vi "LaserMaster.vi"() -> ()   [LabVIEW 2013]
uses:
  <vilib>/Instr/_visa.llb/VISA Configure Serial Port (Instr).vi
  <vilib>/Utility/file.llb/Write To Spreadsheet File (string).vi
panel:
  out "Humidity Threshold":dbl
  in  "Power (mW) 2":dbl format="%#.0f"
  out "SavePath":path
  out "Start time":timestamp
  out "Step":dbl
  out "State next step":string
  in  "stop":bool
  out "Query backup List":string[][](array[string])=[["?L", " 0\r"], ["?K", " 0\r"], ["?F", " 0\r"], ["?FH", " 2\r"], ["?SHUTTER", " 0\r"], ["?UF", " 0\r"], ["?PHLDC", " 1\r"], ["?PZTMC", " 0\r"], ["?PZTXC", " 2.24\r"], ["?PZTYC", " 2.14\r"], ["?PHLDP", " 0\r"], ["?PZTMP", " 0\r"], ["?PZTXP", " 2.58\r"], ["?PXTYP", "  Query Error:?PXTYP\r"], ["?PTRK", "  Query Error:?PTRK\r"], ["?MDLK", " 0\r"], ["?PP", " 0.80\r"], ["?TS", " 0\r"], ["?SM", " 1\r"], ["?HM", " 1\r"], ["?VW", " 850\r"], ["?STPRPOS", " 2096\r"], ["?C", " 0.00\r"], ["?D1C", " 0.08\r"], ["?D2C", " -0.43\r"], ["?BT", " 20.07\r"], ["?D1T", " 24.20\r"], ["?D2T", " 24.20\r"], ["?VT", " 20.72\r"], ["?LBOT", " 148.45\r"], ["?ET", " 39.01\r"], ["?D1ST", " 24.20\r"], ["?D2ST", " 24.20\r"], ["?VST", " 30.00\r"], ["?LBOST", " 148.41\r"], ["?EST", " 39.00\r"], ["?D1TD", " 500.12\r"], ["?D2TD", " 464.53\r"], ["?VD", " 0.00\r"], ["?LBOD", " 5358.08\r"], ["?ED", " 2152.46\r"], ["?D1HST", " 21.35\r"], ["?D2HST", " 21.48\r"], ["?LBOH", " 1\r"], ["?LRS", " 2\r"], ["?D1SS", " 1\r"], ["?D2SS", " 1\r"], ["?VSS", " 0\r"], ["?LBOSS", " 1\r"], ["?ESS", " 1\r"], ["?D1H", "  351.54\r"], ["?D2H", "  351.52\r"], ["?HH", " 37\r"], ["?D1V", " 0.19\r"], ["?D2V", " 0.18\r"], ["?SV", " 8.26,8.26,9.57\r"], ["?MB", "  Query Error:?MB\r"], ["?PI", " 2BC\r"], ["?BV", " 13.24\r"], ["?AMDLK", " 1\r"], ["?PZTS", "  Query Error:?PZTS\r"], ["?TMAX", " 1080\r"], ["?TMIN", " 680\r"], ["?ALIGN", " 0\r"], ["?ALIGNP", " 250\r"], ["?ALIGNW", " 730\r"], ["?LFP", " 0\r"], ["?PZTXCM", " 8.11\r"], ["?PZTXCP", " -10.30\r"], ["?PZTXPM", " 8.11\r"], ["?PZTXPP", " 3.06\r"], ["?PZTYCM", " 8.11\r"], ["?PZTYCP", " -14.28\r"], ["?PZTYPM", " 8.11\r"], ["?PZTYPP", " 11.74\r"], ["?RH", " 0\r"], ["?SN", " 9571\r"], ["?ST", " Standby\r"], ["?GDDCURVE", " 0\r"], ["?GDD", " 0\r"], ["?GDDCURVEN", " ZERO\r"], ["?CURVEN", " OUT OF RANGE\r"], ["?COMP", " 1\r"], ["?HMCOMP", " 1\r"], ["?GDDMAX", " 17333\r"], ["?GDDMIN", "0"]]
  out "Laser Info":i32
  out "Shutter off time":dbl
  out "Quiting":dbl
  out "Backuper state":string
  in  "Tab Control":T1(tab)
  in  "Auto":bool
  out "Baseplate Temp (C)":dbl(slide) scale=20.0..40.0
  in  "Dither hold":bool
  in  "Shutter":bool
  in  "Lock":bool
  out "Laser Status":bool
  out "Power (mW)":dbl(knob) scale=0.0..5000.0
  out "Walking":bool
  out "Sleeping":bool
  out "ModeLocked":bool
  out "Backing up":bool
  in  "Wavelength":dbl
  in  "GDD":dbl
  in  "Align":bool
  in  "QUIT":bool
  out "Max":string
  in  "Dither auto":dbl=120.0
  in  "Dither timer":dbl=5.0
  out "Faults":string
  in  "Home motor":bool
  in  "Optimize":bool
  in  "WV Walk":bool
  in  "Auto-Standby\nTime (min)":dbl=120.0
  in  "Sleep":bool
  in  "Backup":bool
  in  "Auto-Backup \nIdle Time (min)":dbl=30.0
  out "Operating Status":string
  out "Tunning Status":i32
  out "Idle Time":dbl format="%.1f"
  out "Laser On Time":dbl format="%#.1f"
  in  "Laser Control":bool
  in  "Command Line":string
  out "Laser Response":string
  in  "Refresh":bool
  out "Query List":string[][](array[string])
  out "queue #":i32
  # "LASER"
  # "LASER fine-tune"
  # "BACKUP"
  # "Timers"
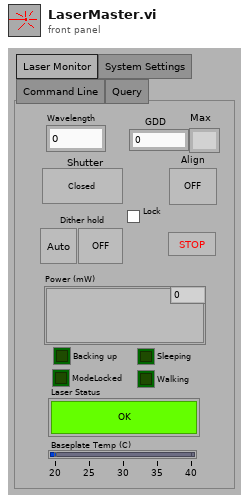
[diagram p1: front panel]
types:
  T1 = enum32{"Laser Monitor", "System Settings", "Command Line", "Query"}
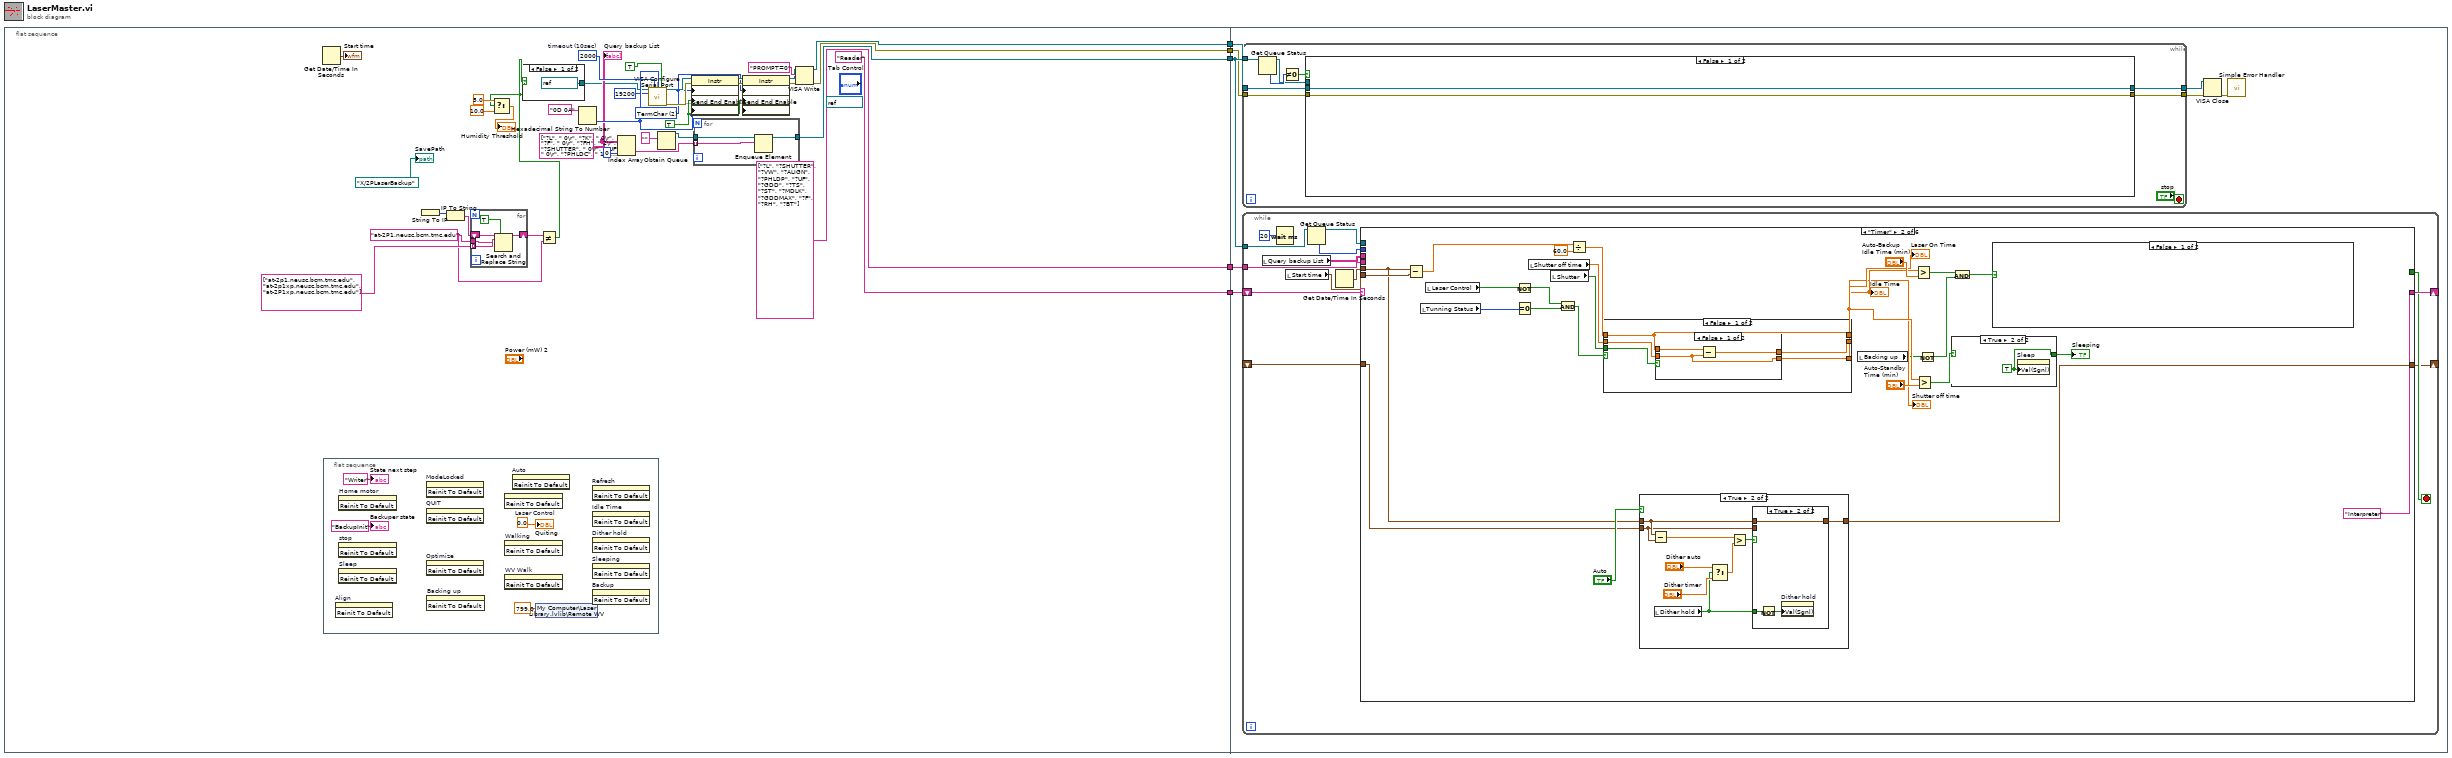
[diagram p0: block diagram]
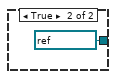
[diagram p2: hidden frame]
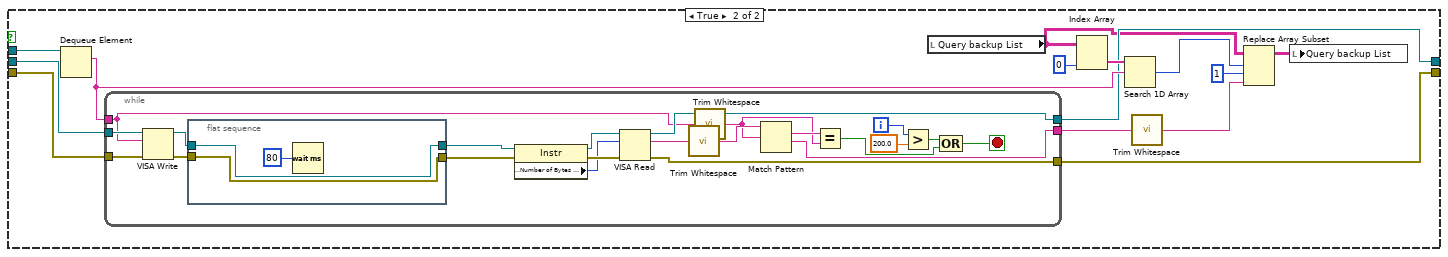
[diagram p3: hidden frame]
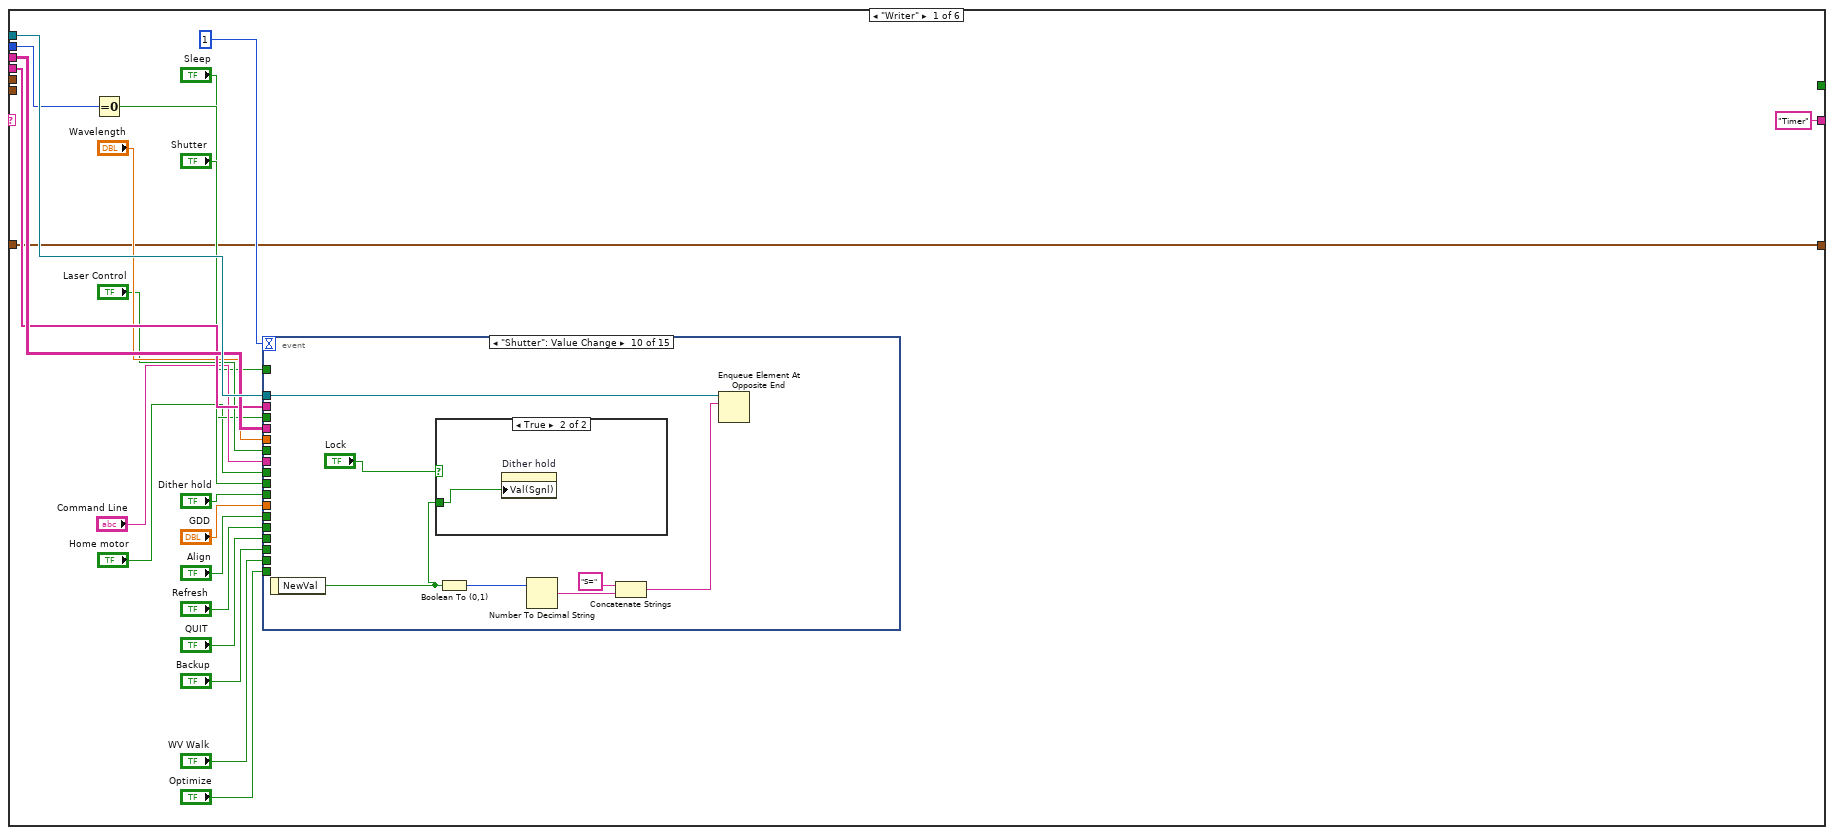
[diagram p4: hidden frame]
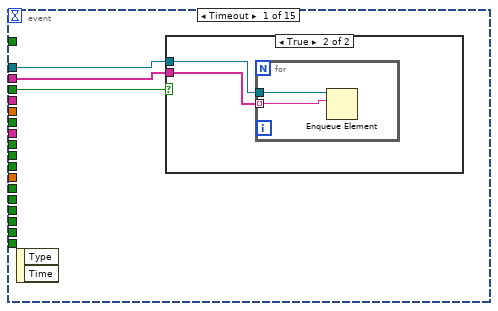
[diagram p5: hidden frame]
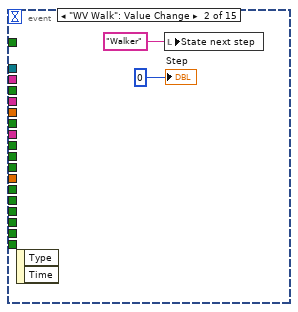
[diagram p7: hidden frame]
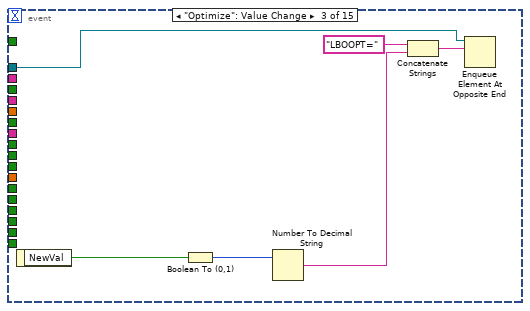
[diagram p8: hidden frame]
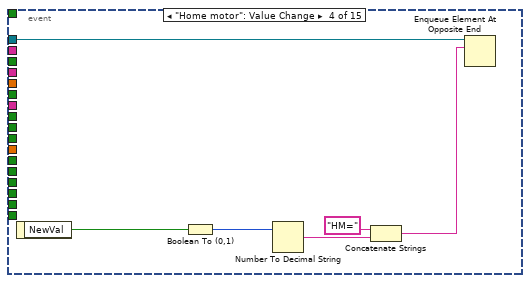
[diagram p9: hidden frame]
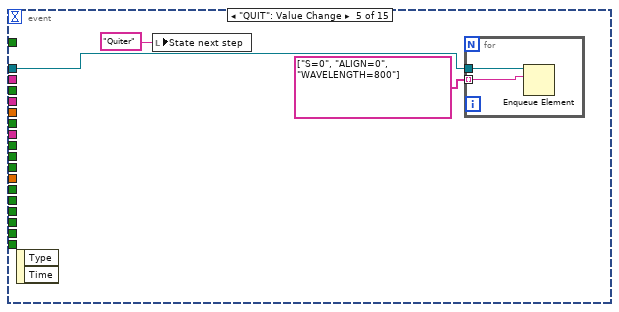
[diagram p10: hidden frame]
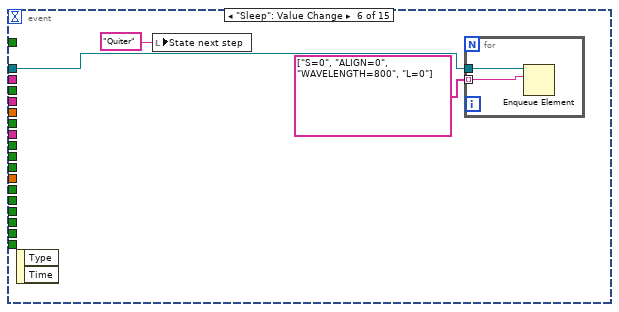
[diagram p11: hidden frame]
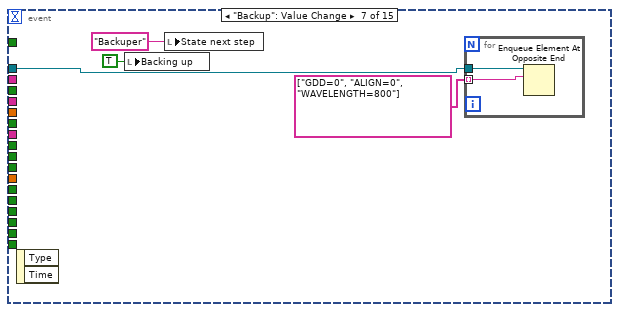
[diagram p12: hidden frame]
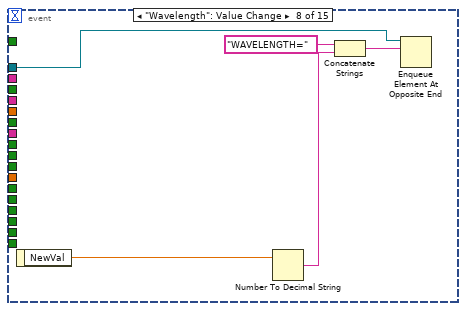
[diagram p13: hidden frame]
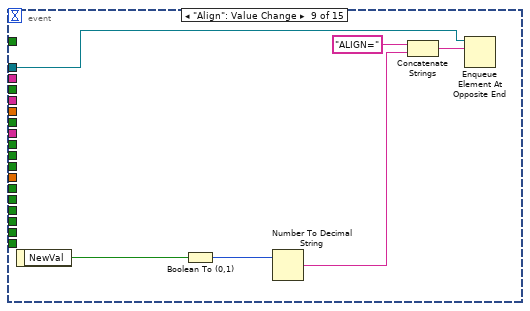
[diagram p14: hidden frame]
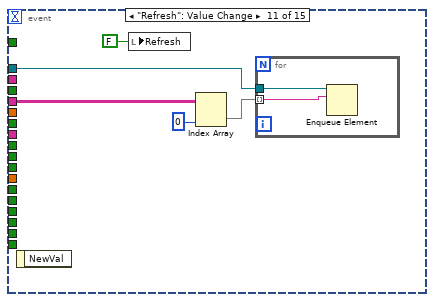
[diagram p16: hidden frame]
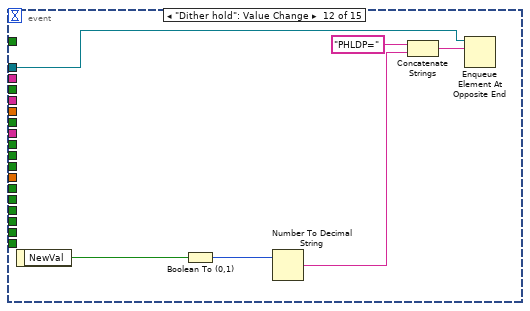
[diagram p17: hidden frame]
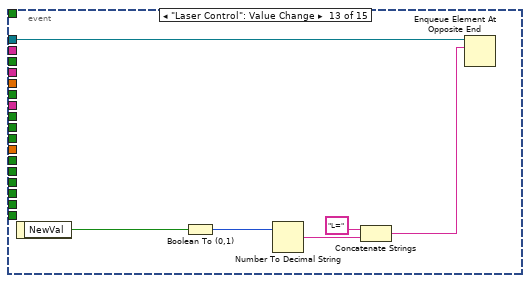
[diagram p18: hidden frame]
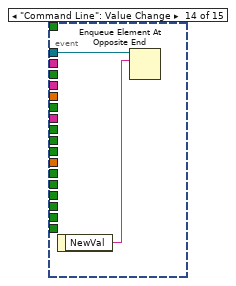
[diagram p19: hidden frame]
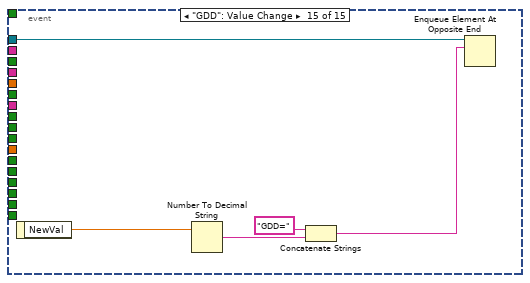
[diagram p20: hidden frame]
diagram:
  n1 = flat-sequence {
    tunnel: [w30] -> w5
    tunnel: [w29] -> w4
    tunnel: [w20] -> w3
    tunnel: [string[] ["?L", "?SHUTTER", "?VW", "?ALIGN", "?PHLDP", "?UF", "?GDD", "?TS", "?ST", "?MDLK", "?GDDMAX", "?F", "?RH", "?BT"]] -> w2
    tunnel: ["Reader"] -> w1
    tunnel: w5 -> [w59]
    tunnel: w4 -> [w56]
    tunnel: w3 -> [w60]
    tunnel: w2 -> [w62]
    tunnel: w1 -> [w61]
    frame #0 {
      w6 = "at-2P1.neusc.bcm.tmc.edu"
      (unwired) refnum<visa-resource-name> "COM1" ("VISA resource name")
      w19 = string[][] [["?L", " 0\r"], ["?K", " 0\r"], ["?F", " 0\r"], ["?FH", " 2\r"], ["?SHUTTER", " 0\r"], ["?UF", " 0\r"], ["?PHLDC", " 1\r"], ["?PZTMC", " 0\r"], ["?PZTXC", " 2.24\r"], ["?PZTYC", " 2.14\r"], ["?PHLDP", " 0\r"], ["?PZTMP", " 0\r"], ["?PZTXP", " 2.58\r"], ["?PXTYP", "  Query Error:?PXTYP\r"], ["?PTRK", "  Query Error:?PTRK\r"], ["?MDLK", " 0\r"], ["?PP", " 0.80\r"], ["?TS", " 0\r"], ["?SM", " 1\r"], ["?HM", " 1\r"], ["?VW", " 850\r"], ["?STPRPOS", " 2096\r"], ["?C", " 0.00\r"], ["?D1C", " 0.08\r"], ["?D2C", " -0.43\r"], ["?BT", " 20.07\r"], ["?D1T", " 24.20\r"], ["?D2T", " 24.20\r"], ["?VT", " 20.72\r"], ["?LBOT", " 148.45\r"], ["?ET", " 39.01\r"], ["?D1ST", " 24.20\r"], ["?D2ST", " 24.20\r"], ["?VST", " 30.00\r"], ["?LBOST", " 148.41\r"], ["?EST", " 39.00\r"], ["?D1TD", " 500.12\r"], ["?D2TD", " 464.53\r"], ["?VD", " 0.00\r"], ["?LBOD", " 5358.08\r"], ["?ED", " 2152.46\r"], ["?D1HST", " 21.35\r"], ["?D2HST", " 21.48\r"], ["?LBOH", " 1\r"], ["?LRS", " 2\r"], ["?D1SS", " 1\r"], ["?D2SS", " 1\r"], ["?VSS", " 0\r"], ["?LBOSS", " 1\r"], ["?ESS", " 1\r"], ["?D1H", "  351.54\r"], ["?D2H", "  351.52\r"], ["?HH", " 37\r"], ["?D1V", " 0.19\r"], ["?D2V", " 0.18\r"], ["?SV", " 8.26,8.26,9.57\r"], ["?MB", "  Query Error:?MB\r"], ["?PI", " 2BC\r"], ["?BV", " 13.24\r"], ["?AMDLK", " 1\r"], ["?PZTS", "  Query Error:?PZTS\r"], ["?TMAX", " 1080\r"], ["?TMIN", " 680\r"], ["?ALIGN", " 0\r"], ["?ALIGNP", " 250\r"], ["?ALIGNW", " 730\r"], ["?LFP", " 0\r"], ["?PZTXCM", " 8.11\r"], ["?PZTXCP", " -10.30\r"], ["?PZTXPM", " 8.11\r"], ["?PZTXPP", " 3.06\r"], ["?PZTYCM", " 8.11\r"], ["?PZTYCP", " -14.28\r"], ["?PZTYPM", " 8.11\r"], ["?PZTYPP", " 11.74\r"], ["?RH", " 0\r"], ["?SN", " 9571\r"], ["?ST", " Standby\r"], ["?GDDCURVE", " 0\r"], ["?GDD", " 0\r"], ["?GDDCURVEN", " ZERO\r"], ["?CURVEN", " OUT OF RANGE\r"], ["?COMP", " 1\r"], ["?HMCOMP", " 1\r"], ["?GDDMAX", " 17333\r"], ["?GDDMIN", "0"]] ("Query backup List")
      w33 = TRUE ("Message Based Settings:Send End Enable")
      w34 = u16 2 items=["None", "LastBit", "TermChar", "Break"] ("Serial Settings:Serial End Mode for Writes")
      w41 = u32 2000  # timeout (10sec)
      n2 = Get Date/Time In Seconds() -> (seconds since 1Jan1904=→"Start time":timestamp)
      n3 = flat-sequence {
        frame #0 {
          n4 = invoke on="Align" class="Bool (strict)" method="Reinit To Default"() -> ()  [unwired: 3 in, 3 out]
          n5 = invoke on="Home motor" class="Bool" method="Reinit To Default"() -> ()  [unwired: 3 in, 3 out]
          n6 = invoke on="stop" class="Bool (strict)" method="Reinit To Default"() -> ()  [unwired: 3 in, 3 out]
          n7 = invoke on="Sleep" class="Bool (strict)" method="Reinit To Default"() -> ()  [unwired: 3 in, 3 out]
          n8 = invoke on="ModeLocked" class="Bool (strict)" method="Reinit To Default"() -> ()  [unwired: 3 in, 3 out]
          n9 = invoke on="QUIT" class="Bool (strict)" method="Reinit To Default"() -> ()  [unwired: 3 in, 3 out]
          n10 = invoke on="Optimize" class="Bool" method="Reinit To Default"() -> ()  [unwired: 3 in, 3 out]
          n11 = invoke on="Backing up" class="Bool (strict)" method="Reinit To Default"() -> ()  [unwired: 3 in, 3 out]
          n12 = invoke on="Laser Control" class="Bool (strict)" method="Reinit To Default"() -> ()  [unwired: 3 in, 3 out]
          n13 = invoke on="Walking" class="Bool (strict)" method="Reinit To Default"() -> ()  [unwired: 3 in, 3 out]
          n14 = invoke on="WV Walk" class="Bool (strict)" method="Reinit To Default"() -> ()  [unwired: 3 in, 3 out]
          n15 = invoke on="Auto" class="Bool (strict)" method="Reinit To Default"() -> ()  [unwired: 3 in, 3 out]
          n16 = shared-variable "My Computer\\Laser Library.lvlib\\Remote WV"(799.0 ("Remote WV")) -> ()  [unwired: 1 in, 1 out]
          n17 = invoke on="Refresh" class="Bool (strict)" method="Reinit To Default"() -> ()  [unwired: 3 in, 3 out]
          n18 = invoke on="Idle Time" class="DigNum (strict)" method="Reinit To Default"() -> ()  [unwired: 3 in, 3 out]
          n19 = invoke on="Dither hold" class="Bool (strict)" method="Reinit To Default"() -> ()  [unwired: 3 in, 3 out]
          n20 = invoke on="Sleeping" class="Bool (strict)" method="Reinit To Default"() -> ()  [unwired: 3 in, 3 out]
          n21 = invoke on="Backup" class="Bool (strict)" method="Reinit To Default"() -> ()  [unwired: 3 in, 3 out]
          "Backuper state" <- "BackupInit"
          "Quiting" <- 0.0 ("Quiting")
          "State next step" <- "Writer"
        }
      }
      n22 = String To IP() -> (0:w11:u32)  [unwired: 1 in]
      n23 = IP To String(2:w11) -> (0:w10:string)  [unwired: 1 in]
      n24 = for {
        tunnel: string[] ["at-2p1.neusc.bcm.tmc.edu", "at-2p1xp.neusc.bcm.tmc.edu", "at-2P1xp.neusc.bcm.tmc.edu"] -> [w46] mode=indexing
        shift-right: [w44] -> w9
        shift-left: w10 -> [w45]
        tunnel: w6 -> [w43]
        n25 = Search and Replace String(replace all?=TRUE ("replace all? (F)"), input string=w45, search string=w46, replace string=w43) -> (result string=w44:string)  [unwired: 4 in, 3 out]
      }
      n26 = Not Equal?(x=w9, y=w6) -> (x != y?=w8:bool)
      n27 = Select(t=5.0, s=w8, f=10.0) -> (s? t:f=→"Humidity Threshold":dbl)
      n28 = case shown="False" w8 {
        tunnel: [refnum<visa-resource-name> "COM1" ("VISA resource name") refnum<visa-resource-name> "COM6" ("VISA resource name")] -> w16
        frame False {
        }
        frame True {
        }
      }
      n29 = Hexadecimal String To Number(string="0D 0A") -> (number=w32:u32)  [unwired: 2 in, 1 out]
      n30 = Index Array(array=w19, index (col)=0 ("disabled index (col)")) -> (element=w22:string[])  [unwired: 1 in]
      n31 = call-poly "VISA Configure Serial Port"("VISA resource name"=w16, "timeout (10sec)"=w41, "termination char\n(0xA = '\\n' = LF)"=w32, "Enable Termination\nChar (T)"=TRUE ("Enable Termination\nChar (T)"), "baud rate (9600)"=u32 19200) -> ("VISA resource name out"=w38:refnum<visa-resource-name>, "error out"=w37:errorcluster)  [unwired: 5 in, 4 out]
      n32 = Obtain Queue(element data type="") -> (queue out=w24:refnum<queue>)  [unwired: 4 in, 2 out]
      n33 = property class="Instr"(reference=w38, error in=w37, "Serial Settings:End Mode for Writes"=w34, "Message Based Settings:Send End Enable"=w33, "Message Based Settings:Termination Character"=w32) -> (reference out=w36:refnum<visa-resource-name>, error out=w35:errorcluster)
      n34 = for {
        tunnel: w24 -> [w55]
        tunnel: w22 -> [w54] mode=indexing
        tunnel: [w53] -> w20
        n35 = Enqueue Element(queue=w55, element=w54) -> (queue out=w53:refnum<queue>)  [unwired: 2 in, 2 out]
      }
      n36 = property class="Instr"(reference=w36, error in=w35, "Serial Settings:End Mode for Writes"=w34, "Message Based Settings:Send End Enable"=w33, "Message Based Settings:Termination Character"=w32) -> (reference out=w27:refnum<visa-resource-name>, error out=w26:errorcluster)
      n37 = VISA Write(VISA resource name=w27, write buffer="PROMPT=0", error in (no error)=w26) -> (VISA resource name out=w30:refnum<visa-resource-name>, error out=w29:errorcluster)  [unwired: 1 out]
      "Query backup List" <- w19
      "SavePath" <- path "X:/2PLaserBackup"
    }
    frame #1 {
      n38 = while {
        tunnel: w60 -> [w67]
        tunnel: w59 -> [w72]
        tunnel: [w71] -> w58
        tunnel: [w70] -> w57
        tunnel: w56 -> [w69]
        stop <- "stop" stop-if-true
        n39 = Get Queue Status(queue=w67) -> (queue out=w64:refnum<queue>, # elements in queue=w66:i32)  [unwired: 2 in, 6 out]
        n40 = Not Equal To 0?(x=w66) -> (x != 0?=w65:bool)
        n41 = case shown="False" w65 {
          tunnel: w64 -> [_ w81]
          tunnel: w72 -> [w74 w80]
          tunnel: [w74 w79] -> w71
          tunnel: [w73 w78] -> w70
          tunnel: w69 -> [w73 w77]
          frame False {
          }
          frame True {
            n42 = Dequeue Element(queue=w81) -> (element=w83:string)  [unwired: 2 in, 3 out]
            n43 = while {
              tunnel: w80 -> [w110]
              tunnel: w77 -> [w109]
              tunnel: [w108] -> w79
              tunnel: [w107] -> w78
              tunnel: w83 -> [w95]
              tunnel: [w103] -> w84
              i -> [w93]
              stop <- w90 stop-if-true
              n44 = VISA Write(VISA resource name=w110, write buffer=w95, error in (no error)=w109) -> (VISA resource name out=w101:refnum<visa-resource-name>, error out=w98:errorcluster)  [unwired: 1 out]
              n45 = flat-sequence {
                tunnel: [w113] -> w100
                tunnel: w101 -> [w113]
                tunnel: w98 -> [w112]
                tunnel: [w112] -> w99
                frame #0 {
                  n46 = Wait (ms)(milliseconds to wait=u32 80) -> ()  [unwired: 1 out]
                }
              }
              n47 = property class="Instr"(reference=w100, error in=w99) -> (reference out=w106:refnum<visa-resource-name>, error out=w105:errorcluster, "Serial Settings:Number of Bytes at Serial Port"=w104:u32)
              n48 = VISA Read(VISA resource name=w106, byte count=w104, error in (no error)=w105) -> (VISA resource name out=w108:refnum<visa-resource-name>, read buffer=w97:string, error out=w107:errorcluster)  [unwired: 1 out]
              n49 = call <vilib>:"Trim Whitespace.vi"("string"=w97) -> ("trimmed string"=w96:string)  [unwired: 1 in]
              n50 = call <vilib>:"Trim Whitespace.vi"("string"=w95) -> ("trimmed string"=w89:string)  [unwired: 1 in]
              n51 = Match Pattern(string=w96, regular expression=w89) -> (match substring=w102:string, after substring=w103:string)  [unwired: 1 in, 2 out]
              n52 = Equal?(x=w102, y=w89) -> (x = y?=w91:bool)
              n53 = Greater?(x=w93, y=200.0) -> (0:w92:bool)
              n54 = Compound Arithmetic op=OR(w92, w91) -> (w90:bool)
            }
            n55 = local read "Query backup List"() -> (w76:string[][])
            n56 = Index Array(array=w76, index (col)=0 ("index (row)")) -> (element=w87:string[])  [unwired: 1 in]
            n57 = Search 1D Array(1D array=w87, element=w83) -> (index of element=w85:i32)  [unwired: 1 in]
            n58 = call <vilib>:"Trim Whitespace.vi"("string"=w84) -> ("trimmed string"=w82:string)  [unwired: 1 in]
            n59 = Replace Array Subset(array=w76, new element=w82, index (row)=w85, index (col)=1 ("disabled index (col)")) -> (w75:string[][])
            n60 = local write "Query backup List"(w75) -> ()
          }
        }
      }
      n61 = while {
        tunnel: w60 -> [w123]
        tunnel: w62 -> [w124]
        shift-right: [w125] -> _
        shift-left: w61 -> [w126]
        shift-right: [w115] -> _
        shift-left: _ -> [w114]
        stop <- w120 stop-if-true
        n62 = local read "Query backup List"() -> (w122:string[][])
        n63 = Wait (ms)(milliseconds to wait=u32 20) -> ()  [unwired: 1 out]
        n64 = local read "Start time"() -> (w116:timestamp)
        n65 = Get Queue Status(queue=w123) -> (queue out=w119:refnum<queue>, # elements in queue=w118:i32)  [unwired: 2 in, 6 out]
        n66 = Get Date/Time In Seconds() -> (seconds since 1Jan1904=w117:timestamp)
        n67 = case shown="\"Timer\"" w126 {
          tunnel: w119 -> [w148 _ _ _ _ _]
          tunnel: w122 -> [w147 _ w301 _ w456 _]
          tunnel: w124 -> [w146 _ w302 _ _ _]
          tunnel: ["Timer" "Interpreter" w300 "Writer" "Writer" w482] -> w125
          tunnel: w118 -> [w145 _ w299 _ _ w484]
          tunnel: [_ _ _ _ _ w481] -> w120
          tunnel: w117 -> [_ w232 _ _ _ _]
          tunnel: w116 -> [_ w236 _ _ _ _]
          tunnel: [w127 w233 w298 w438 w453 w480] -> w115
          tunnel: w114 -> [w127 w231 w298 w438 w453 w480]
          frame "Writer" {
            n68 = Equal To 0?(x=w145) -> (x = 0?=w133:bool)
            n69 = event shown="[9] \"Shutter\": Value Change" {
              selector: _ -> [_ _ _ _ _ _ _ _ _ _ _ _ _ _ _]
              dyn-events: _ -> [_ _ _ _ _ _ _ _ _ _ _ _ _ _ _]
              timeout: 1 -> [_ _ _ _ _ _ _ _ _ _ _ _ _ _ _]
              tunnel: w148 -> [w151 _ w158 w165 w171 w175 w182 w187 w192 w199 w206 w213 w218 w225 w227]
              tunnel: "Shutter" -> [_ _ _ _ _ _ _ _ _ _ _ _ _ _ _]
              tunnel: "Dither hold" -> [_ _ _ _ _ _ _ _ _ _ _ _ _ _ _]
              tunnel: "GDD" -> [_ _ _ _ _ _ _ _ _ _ _ _ _ _ _]
              tunnel: "Align" -> [_ _ _ _ _ _ _ _ _ _ _ _ _ _ _]
              tunnel: "Wavelength" -> [_ _ _ _ _ _ _ _ _ _ _ _ _ _ _]
              tunnel: "Laser Control" -> [_ _ _ _ _ _ _ _ _ _ _ _ _ _ _]
              tunnel: "Command Line" -> [_ _ _ _ _ _ _ _ _ _ _ _ _ _ _]
              tunnel: w147 -> [_ _ _ _ _ _ _ _ _ _ w205 _ _ _ _]
              tunnel: "Refresh" -> [_ _ _ _ _ _ _ _ _ _ _ _ _ _ _]
              tunnel: w146 -> [w150 _ _ _ _ _ _ _ _ _ _ _ _ _ _]
              tunnel: "QUIT" -> [_ _ _ _ _ _ _ _ _ _ _ _ _ _ _]
              tunnel: "Backup" -> [_ _ _ _ _ _ _ _ _ _ _ _ _ _ _]
              tunnel: w133 -> [w149 _ _ _ _ _ _ _ _ _ _ _ _ _ _]
              tunnel: "WV Walk" -> [_ _ _ _ _ _ _ _ _ _ _ _ _ _ _]
              tunnel: "Optimize" -> [_ _ _ _ _ _ _ _ _ _ _ _ _ _ _]
              tunnel: "Home motor" -> [_ _ _ _ _ _ _ _ _ _ _ _ _ _ _]
              tunnel: "Sleep" -> [_ _ _ _ _ _ _ _ _ _ _ _ _ _ _]
              event Timeout {
                n70 = event-data() -> ()  [unwired: 1 in, 2 out]
                n71 = case shown="True" w149 {
                  tunnel: w151 -> [_ w153]
                  tunnel: w150 -> [_ w152]
                  frame False {
                  }
                  frame True {
                    n72 = for {
                      tunnel: w153 -> [w155]
                      tunnel: w152 -> [w154] mode=indexing
                      n73 = Enqueue Element(queue=w155, element=w154) -> ()  [unwired: 2 in, 3 out]
                    }
                  }
                }
              }
              event "WV Walk": Value Change {
                n74 = event-data() -> ()  [unwired: 1 in, 2 out]
                n75 = local write "State next step"("Walker") -> ()
                "Step" <- 0
              }
              event "Optimize": Value Change {
                n76 = event-data() -> ("NewVal"=w159:bool)  [unwired: 1 in]
                n77 = Boolean To (0,1)(Boolean=w159) -> (0, 1=w162:i16)
                n78 = Number To Decimal String(number=w162) -> (decimal integer string=w163:string)  [unwired: 1 in]
                n79 = Concatenate Strings("LBOOPT=", w163) -> (w160:string)
                n80 = Enqueue Element At Opposite End(queue=w158, element=w160) -> ()  [unwired: 2 in, 3 out]
              }
              event "Home motor": Value Change {
                n81 = event-data() -> ("NewVal"=w164:bool)  [unwired: 1 in]
                n82 = Boolean To (0,1)(Boolean=w164) -> (0, 1=w168:i16)
                n83 = Number To Decimal String(number=w168) -> (decimal integer string=w169:string)  [unwired: 1 in]
                n84 = Concatenate Strings("HM=", w169) -> (w166:string)
                n85 = Enqueue Element At Opposite End(queue=w165, element=w166) -> ()  [unwired: 2 in, 3 out]
              }
              event "QUIT": Value Change {
                n86 = event-data() -> ()  [unwired: 1 in, 2 out]
                n87 = local write "State next step"("Quiter") -> ()
                n88 = for {
                  tunnel: w171 -> [w174]
                  tunnel: string[] ["S=0", "ALIGN=0", "WAVELENGTH=800"] -> [w173] mode=indexing
                  n89 = Enqueue Element(queue=w174, element=w173) -> ()  [unwired: 2 in, 3 out]
                }
              }
              event "Sleep": Value Change {
                n90 = event-data() -> ()  [unwired: 1 in, 2 out]
                n91 = local write "State next step"("Quiter") -> ()
                n92 = for {
                  tunnel: w175 -> [w179]
                  tunnel: string[] ["S=0", "ALIGN=0", "WAVELENGTH=800", "L=0"] -> [w178] mode=indexing
                  n93 = Enqueue Element(queue=w179, element=w178) -> ()  [unwired: 2 in, 3 out]
                }
              }
              event "Backup": Value Change {
                n94 = event-data() -> ()  [unwired: 1 in, 2 out]
                n95 = local write "Backing up"(TRUE ("Backing up ...")) -> ()
                n96 = local write "State next step"("Backuper") -> ()
                n97 = for {
                  tunnel: string[] ["GDD=0", "ALIGN=0", "WAVELENGTH=800"] -> [w185] mode=indexing
                  tunnel: w182 -> [w184]
                  n98 = Enqueue Element At Opposite End(queue=w184, element=w185) -> ()  [unwired: 2 in, 3 out]
                }
              }
              event "Wavelength": Value Change {
                n99 = event-data() -> ("NewVal"=w186:dbl)  [unwired: 1 in]
                n100 = Number To Decimal String(number=w186) -> (decimal integer string=w189:string)  [unwired: 1 in]
                n101 = Concatenate Strings("WAVELENGTH=", w189) -> (w190:string)
                n102 = Enqueue Element At Opposite End(queue=w187, element=w190) -> ()  [unwired: 2 in, 3 out]
              }
              event "Align": Value Change {
                n103 = event-data() -> ("NewVal"=w191:bool)  [unwired: 1 in]
                n104 = Boolean To (0,1)(Boolean=w191) -> (0, 1=w195:i16)
                n105 = Number To Decimal String(number=w195) -> (decimal integer string=w196:string)  [unwired: 1 in]
                n106 = Concatenate Strings("ALIGN=", w196) -> (w193:string)
                n107 = Enqueue Element At Opposite End(queue=w192, element=w193) -> ()  [unwired: 2 in, 3 out]
              }
              event "Shutter": Value Change {
                n108 = event-data() -> ("NewVal"=w197:bool)  [unwired: 1 in]
                n109 = case shown="True" "Lock" {
                  tunnel: w197 -> [_ w204]
                  frame False {
                  }
                  frame True {
                    n110 = property on="Dither hold" class="Bool (strict)"("Val(Sgnl)"=w204) -> ()  [unwired: 2 in, 2 out]
                  }
                }
                n111 = Boolean To (0,1)(Boolean=w197) -> (0, 1=w202:i16)
                n112 = Number To Decimal String(number=w202) -> (decimal integer string=w203:string)  [unwired: 1 in]
                n113 = Concatenate Strings("S=", w203) -> (w200:string)
                n114 = Enqueue Element At Opposite End(queue=w199, element=w200) -> ()  [unwired: 2 in, 3 out]
              }
              event "Refresh": Value Change {
                n115 = event-data() -> ()  [unwired: 1 in, 1 out]
                n116 = local write "Refresh"(FALSE ("Backup")) -> ()
                n117 = Index Array(array=w205, index (col)=0 ("disabled index (col)")) -> (element=w208:string[])  [unwired: 1 in]
                n118 = for {
                  tunnel: w206 -> [w211]
                  tunnel: w208 -> [w210] mode=indexing
                  n119 = Enqueue Element(queue=w211, element=w210) -> ()  [unwired: 2 in, 3 out]
                }
              }
              event "Dither hold": Value Change {
                n120 = event-data() -> ("NewVal"=w212:bool)  [unwired: 1 in]
                n121 = Boolean To (0,1)(Boolean=w212) -> (0, 1=w216:i16)
                n122 = Number To Decimal String(number=w216) -> (decimal integer string=w217:string)  [unwired: 1 in]
                n123 = Concatenate Strings("PHLDP=", w217) -> (w214:string)
                n124 = Enqueue Element At Opposite End(queue=w213, element=w214) -> ()  [unwired: 2 in, 3 out]
              }
              event "Laser Control": Value Change {
                n125 = event-data() -> ("NewVal"=w219:bool)  [unwired: 1 in]
                n126 = Boolean To (0,1)(Boolean=w219) -> (0, 1=w222:i16)
                n127 = Number To Decimal String(number=w222) -> (decimal integer string=w223:string)  [unwired: 1 in]
                n128 = Concatenate Strings("L=", w223) -> (w220:string)
                n129 = Enqueue Element At Opposite End(queue=w218, element=w220) -> ()  [unwired: 2 in, 3 out]
              }
              event "Command Line": Value Change {
                n130 = event-data() -> ("NewVal"=w224:string)  [unwired: 1 in]
                n131 = Enqueue Element At Opposite End(queue=w225, element=w224) -> ()  [unwired: 2 in, 3 out]
              }
              event "GDD": Value Change {
                n132 = event-data() -> ("NewVal"=w226:dbl)  [unwired: 1 in]
                n133 = Number To Decimal String(number=w226) -> (decimal integer string=w229:string)  [unwired: 1 in]
                n134 = Concatenate Strings("GDD=", w229) -> (w230:string)
                n135 = Enqueue Element At Opposite End(queue=w227, element=w230) -> ()  [unwired: 2 in, 3 out]
              }
            }
          }
          frame "Timer" {
            n136 = Subtract(x=w232, y=w236) -> (x-y=w239:dbl)
            n137 = local read "Tunning Status"() -> (w256:i32)
            n138 = local read "Laser Control"() -> (w255:bool)
            n139 = Not(x=w255) -> (.not. x?=w251:bool)
            n140 = Equal To 0?(x=w256) -> (x = 0?=w250:bool)
            n141 = local read "Shutter off time"() -> (w246:dbl)
            n142 = local read "Shutter"() -> (w247:bool)
            n143 = And(x=w251, y=w250) -> (x .and. y?=w252:bool)
            n144 = Divide(x=w239, y=60.0 ("x")) -> (x/y=w237:dbl)
            n145 = case shown="False" w252 {
              tunnel: [w272 w283] -> w249
              tunnel: [w276 w283] -> w248
              tunnel: w247 -> [w275 _]
              tunnel: w246 -> [w274 _]
              tunnel: [w273 w283] -> w245
              tunnel: w237 -> [w272 _]
              frame False {
                n146 = case shown="False" w275 {
                  tunnel: [w279 0] -> w276
                  tunnel: w272 -> [w278 w280]
                  tunnel: w274 -> [w277 _]
                  tunnel: [w277 w280] -> w273
                  frame False {
                    n147 = Subtract(x=w278, y=w277) -> (x-y=w279:dbl)
                  }
                  frame True {
                  }
                }
              }
              frame True {
                w283 = 0
                n148 = Get Date/Time In Seconds() -> (seconds since 1Jan1904=w282:timestamp)
                n149 = local write "Start time"(w282) -> ()
              }
            }
            "Laser On Time" <- w249
            "Idle Time" <- w248
            "Shutter off time" <- w245
            n150 = case shown="True" "Auto" {
              tunnel: w232 -> [w258 w265]
              tunnel: [w258 w264] -> w233
              tunnel: w231 -> [_ w263]
              frame False {
              }
              frame True {
                n151 = Subtract(x=w265, y=w263) -> (x-y=w267:dbl)
                n152 = local read "Dither hold"() -> (w259:bool)
                n153 = Select(t="Dither auto", s=w259, f="Dither timer") -> (s? t:f=w260:dbl)
                n154 = Greater?(x=w267, y=w260) -> (0:w266:bool)
                n155 = case shown="True" w266 {
                  tunnel: w265 -> [_ w271]
                  tunnel: [w268 w271] -> w264
                  tunnel: w263 -> [w268 _]
                  tunnel: w259 -> [_ w270]
                  frame False {
                  }
                  frame True {
                    n156 = Not(x=w270) -> (.not. x?=w269:bool)
                    n157 = property on="Dither hold" class="Bool (strict)"("Val(Sgnl)"=w269) -> ()  [unwired: 2 in, 2 out]
                  }
                }
              }
            }
            n158 = local read "Backing up"() -> (w240:bool)
            n159 = Greater?(x=w248, y="Auto-Backup \nIdle Time (min)") -> (0:w243:bool)
            n160 = Greater?(x=w248, y="Auto-Standby\nTime (min)") -> (0:w235:bool)
            n161 = Not(x=w240) -> (.not. x?=w242:bool)
            n162 = case shown="True" w235 {
              tunnel: [FALSE ("Sleeping") w285] -> w244
              frame False {
              }
              frame True {
                w285 = TRUE
                n163 = property on="Sleep" class="Bool (strict)"("Val(Sgnl)"=w285) -> ()  [unwired: 2 in, 2 out]
              }
            }
            "Sleeping" <- w244
            n164 = And(x=w243, y=w242) -> (x .and. y?=w241:bool)
            n165 = case shown="False" w241 {
              frame False {
              }
              frame True {
                n166 = local read "SavePath"() -> (w286:path)
                n167 = String To IP() -> (0:w290:u32)  [unwired: 1 in]
                n168 = IP To String(2:w290) -> (0:w287:string)  [unwired: 1 in]
                n169 = Get Date/Time In Seconds() -> (seconds since 1Jan1904=w292:timestamp)
                n170 = Format Date/Time String(time format string (%c)="%Y-%m-%d-*", seconds (now)=w292) -> (date/time string=w289:string)  [unwired: 1 in]
                n171 = call "create unique folder.vi"("string"=w287, "path 2"=w286) -> ("path"=w295:path)  [unwired: 9 in]
                n172 = Concatenate Strings(w289, ".csv" ("string")) -> (w294:string)
                n173 = call <vilib>:"Recursive File List.vi"("pattern"=w294, "Folder Path"=w295) -> ("Number of Files"=w296:i32)  [unwired: 5 in, 4 out]
                n174 = Equal To 0?(x=w296) -> (x = 0?=w288:bool)
                n175 = case shown="True" w288 {
                  frame False {
                  }
                  frame True {
                    n176 = property on="Backup" class="Bool (strict)"("Val(Sgnl)"=TRUE) -> ()  [unwired: 2 in, 2 out]
                  }
                }
              }
            }
          }
          frame "Interpreter", Default {
            n177 = stacked-sequence {
              tunnel: w302 -> [_ w318 _ _ _]
              tunnel: w301 -> [w303 w317 _ w403 _]
              frame #0 {
                n178 = Index Array(array=w303, index (col)=0 ("disabled index (col)")) -> (element=w308:string[])  [unwired: 1 in]
                n179 = local read "Command Line"() -> (w307:string)
                n180 = Search 1D Array(1D array=w308, element=w307) -> (index of element=w306:i32)  [unwired: 1 in]
                n181 = Index Array(array=w303, index (row)=w306, index (col)=1 ("disabled index (col)")) -> (element=→"Laser Response":string)
              }
              frame #1 {
                n182 = for {
                  tunnel: w318 -> [w320] mode=indexing
                  tunnel: w317 -> [w321]
                  n183 = Index Array(array=w321, index (col)=0 ("disabled index (col)")) -> (element=w324:string[])  [unwired: 1 in]
                  n184 = Search 1D Array(1D array=w324, element=w320) -> (index of element=w322:i32)  [unwired: 1 in]
                  n185 = Index Array(array=w321, index (row)=w322, index (col)=1 ("disabled index (col)")) -> (element=w319:string)
                  n186 = case shown="\"?RH\"" w320 {
                    tunnel: w319 -> [_ w326 w328 w336 w337 w344 w353 w355 w363 w365 w367 w369 w370 w381 w383]
                    frame "False", Default {
                    }
                    frame "?L" {
                      n187 = Decimal String To Number(string=w326) -> (number=→"Laser Info":i32)  [unwired: 2 in, 1 out]
                    }
                    frame "?SHUTTER" {
                      n188 = Decimal String To Number(string=w328) -> (number=w329:i32)  [unwired: 2 in, 1 out]
                      n189 = local read "Shutter"() -> (w332:bool)
                      n190 = Not Equal To 0?(x=w329) -> (x != 0?=w331:bool)
                      n191 = And(x=w331, y=w332) -> (x .and. y?=w330:bool)
                      n192 = case shown="False" w330 {
                        frame False {
                          n193 = property on="Shutter" class="Bool (strict)"("Colors [4]"=cluster{u32, u32}[] [{12369084, 12369084}, {12369084, 12369084}]) -> ()  [unwired: 2 in, 2 out]
                        }
                        frame True {
                          n194 = property on="Shutter" class="Bool (strict)"("Colors [4]"=cluster{u32, u32}[] [{12369084, 12369084}, {6618880, 6618880}]) -> ()  [unwired: 2 in, 2 out]
                        }
                      }
                    }
                    frame "?VW" {
                      n195 = Decimal String To Number(string=w336) -> (number=w335:i32)  [unwired: 2 in, 1 out]
                      n196 = property on="Wavelength" class="DigNum (strict)"("Value"=w335) -> ()  [unwired: 2 in, 2 out]
                      n197 = shared-variable ".\\Laser Library.lvlib\\WV"(w335) -> ()  [unwired: 1 in, 1 out]
                    }
                    frame "?ALIGN" {
                      n198 = Decimal String To Number(string=w337) -> (number=w338:i32)  [unwired: 2 in, 1 out]
                      n199 = Not Equal To 0?(x=w338) -> (x != 0?=w341:bool)
                      n200 = local read "Align"() -> (w340:bool)
                      n201 = And(x=w341, y=w340) -> (x .and. y?=w339:bool)
                      n202 = case shown="False" w339 {
                        frame False {
                          n203 = property on="Align" class="Bool (strict)"("Colors [4]"=cluster{u32, u32}[] [{12369084, 12369084}, {12369084, 12369084}]) -> ()  [unwired: 2 in, 2 out]
                        }
                        frame True {
                          n204 = property on="Align" class="Bool (strict)"("Colors [4]"=cluster{u32, u32}[] [{12369084, 12369084}, {6618880, 6618880}]) -> ()  [unwired: 2 in, 2 out]
                        }
                      }
                    }
                    frame "?PHLDP" {
                      n205 = Decimal String To Number(string=w344) -> (number=w345:i32)  [unwired: 2 in, 1 out]
                      n206 = Not Equal To 0?(x=w345) -> (x != 0?=w348:bool)
                      n207 = local read "Dither hold"() -> (w346:bool)
                      n208 = And(x=w348, y=w346) -> (x .and. y?=w347:bool)
                      n209 = case shown="False" w347 {
                        frame False {
                          n210 = property on="Dither hold" class="Bool (strict)"("Colors [4]"=cluster{u32, u32}[] [{12369084, 12369084}, {12369084, 12369084}]) -> ()  [unwired: 2 in, 2 out]
                        }
                        frame True {
                          n211 = property on="Dither hold" class="Bool (strict)"("Colors [4]"=cluster{u32, u32}[] [{12369084, 12369084}, {6618880, 6618880}]) -> ()  [unwired: 2 in, 2 out]
                        }
                      }
                    }
                    frame "?UF" {
                      n212 = Decimal String To Number(string=w353) -> (number=w352:i32)  [unwired: 2 in, 1 out]
                      n213 = Round To Nearest(number=w352) -> (nearest integer value=→"Power (mW)":i32)
                    }
                    frame "?GDD" {
                      n214 = Decimal String To Number(string=w355) -> (number=w354:i32)  [unwired: 2 in, 1 out]
                      n215 = property on="GDD" class="DigNum (strict)"("Value"=w354) -> ()  [unwired: 2 in, 2 out]
                      n216 = shared-variable "My Computer\\Laser Library.lvlib\\GDD"(w354) -> ()  [unwired: 1 in, 1 out]
                    }
                    frame "?GDDMAX" {
                      n217 = Decimal String To Number(string=w363) -> (number=w361:i32)  [unwired: 2 in, 1 out]
                      n218 = Divide(x=w361, y=1000.0) -> (x/y=w357:dbl)
                      n219 = Round To Nearest(number=w357) -> (nearest integer value=w356:dbl)
                      n220 = Number To Decimal String(number=w356) -> (decimal integer string=w360:string)  [unwired: 1 in]
                      n221 = Concatenate Strings(w360, "k" ("string")) -> (→"Max":string)
                    }
                    frame "?TS" {
                      n222 = Decimal String To Number(string=w365) -> (number=→"Tunning Status":i32)  [unwired: 2 in, 1 out]
                    }
                    frame "?MDLK" {
                      n223 = Decimal String To Number(string=w367) -> (number=w368:i32)  [unwired: 2 in, 1 out]
                      n224 = Not Equal To 0?(x=w368) -> (x != 0?=→"ModeLocked":bool)
                    }
                    frame "?ST" {
                      "Operating Status" <- w369
                    }
                    frame "?F" {
                      "Faults" <- w370
                    }
                    frame "?RH" {
                      n225 = local read "Humidity Threshold"() -> (w371:dbl)
                      n226 = Decimal String To Number(string=w381) -> (number=w380:i32)  [unwired: 2 in, 1 out]
                      n227 = Greater?(x=w380, y=w371) -> (0:w379:bool)
                      n228 = local read "Operating Status"() -> (w374:string)
                      n229 = local read "Laser Info"() -> (w377:i32)
                      n230 = Select(t=2, s=w379, f=w377) -> (s? t:f=w378:i32)
                      n231 = Concatenate Strings(w374, "\nHigh Humidity") -> (w372:string)
                      n232 = Select(t=w372, s=w379, f=w374) -> (s? t:f=w375:string)
                      n233 = local write "Laser Info"(w378) -> ()
                      n234 = local write "Operating Status"(w375) -> ()
                    }
                    frame "?BT" {
                      n235 = Decimal String To Number(string=w383) -> (number=→"Baseplate Temp (C)":i32)  [unwired: 2 in, 1 out]
                    }
                  }
                }
                n236 = local read "Operating Status"() -> (w313:string)
                n237 = local read "Faults"() -> (w311:string)
                n238 = Decimal String To Number(string=w311) -> (number=w312:i32)  [unwired: 2 in, 1 out]
                n239 = Equal To 0?(x=w312) -> (x = 0?=w310:bool)
                n240 = Select(t=w313, s=w310, f=w311) -> (s? t:f=w314:string)
                n241 = Initialize Array(w314, 4 ("dimension size")) -> (w315:string[])
                n242 = property on="Laser Status" class="Bool (strict)"("Strings [4]"=w315) -> ()  [unwired: 2 in, 2 out]
              }
              frame #2 {
                n243 = local read "Tunning Status"() -> (w384:i32)
                n244 = local read "Laser Info"() -> (w388:i32)
                n245 = Equal To 0?(x=w384) -> (x = 0?=w385:bool)
                n246 = Equal?(x=0, y=w388) -> (x = y?=w386:bool)
                n247 = And(x=w385, y=w386) -> (x .and. y?=w387:bool)
                n248 = Equal?(x=w388, y=2.0) -> (x = y?=w391:bool)
                n249 = case shown="True" w391 {
                  tunnel: w387 -> [w392 _]
                  frame False {
                    n250 = case shown="False" w392 {
                      frame False {
                        w394 = TRUE ("Laser Status")
                        n251 = local read "Operating Status"() -> (w393:string)
                        n252 = local write "Laser Control"(w394) -> ()
                        n253 = local write "Laser Status"(w394) -> ()
                        n254 = Equal?(x=w393, y="OK") -> (x = y?=w395:bool)
                        n255 = case shown="False" w395 {
                          frame False {
                            n256 = property on="Laser Status" class="Bool (strict)"("Colors [4]"=cluster{u32, u32}[] [{16762130, 16762130}, {10441728, 10441728}, {10441728, 10441728}]) -> ()  [unwired: 2 in, 2 out]
                          }
                          frame True {
                            n257 = property on="Laser Status" class="Bool (strict)"("Colors [4]"=cluster{u32, u32}[] [{6618880, 6618880}]) -> ()  [unwired: 2 in, 2 out]
                          }
                        }
                      }
                      frame True {
                        w400 = FALSE
                        n258 = local write "Laser Control"(w400) -> ()
                        n259 = property on="Laser Status" class="Bool (strict)"("Colors [4]"=cluster{u32, u32}[] [{10682272, 10682272}, {12451729, 12451729}]) -> ()  [unwired: 2 in, 2 out]
                        "Laser Status" <- w400
                      }
                    }
                  }
                  frame True {
                    n260 = property on="Laser Status" class="Bool (strict)"("Colors [4]"=cluster{u32, u32}[] [{16723218, 15670016}, {16721170, 16725034}]) -> ()  [unwired: 2 in, 2 out]
                  }
                }
              }
              frame #3 {
                w405 = 2.0 ("y")
                w408 = 30
                n261 = Array Size(array=w403) -> (size(s)=w419:i32[])
                n262 = Index Array(array=w419, index=0) -> (element=w416:i32)
                n263 = Index Array(array=w419, index=1) -> (element=w415:i32)
                n264 = Multiply(x=w416, y=w415) -> (x*y=w413:i32)
                n265 = Divide(x=w413, y=w408) -> (x/y=w414:dbl)
                n266 = Divide(x=w408, y=w405) -> (x/y=w409:dbl)
                n267 = Reshape Array(w403, w413) -> (w412:string[])
                n268 = Subtract(x=w405, y=2.0) -> (x-y=w406:dbl)
                n269 = Round Toward +Infinity(x=w414) -> (ceil(x): smallest int >= x=w407:dbl)
                n270 = Initialize Array("", w409, w406) -> (w410:string[][])
                n271 = for {
                  N: w407 -> [_]
                  tunnel: w408 -> [w433]
                  shift-right: [w431] -> _
                  shift-left: w412 -> [w432]
                  tunnel: w408 -> [w427]
                  tunnel: w405 -> [w420]
                  shift-right: [w421] -> w402
                  shift-left: w410 -> [w423]
                  i -> [w430]
                  n272 = Divide(x=w427, y=w420) -> (x/y=w426:dbl)
                  n273 = Multiply(x=w430, y=w420) -> (x*y=w422:dbl)
                  n274 = Round Toward -Infinity(1:w426) -> (0:w425:dbl)
                  n275 = Split 1D Array(array=w432, index=w433) -> (first subarray=w429:string[], second subarray=w431:string[])
                  n276 = Reshape Array(w429, w425, 2 ("dimension size")) -> (w424:string[][])
                  n277 = Insert Into Array(array=w423, index (col)=w422, new element=w424) -> (w421:string[][])  [unwired: 1 in]
                }
                "Query List" <- w402
              }
              frame #4 {
                n278 = shared-variable ".\\Laser Library.lvlib\\Remote WV"() -> (w434:dbl)  [unwired: 1 in, 1 out]
                n279 = feedback-in #1(w434) -> ()
                n280 = feedback #1(w434) -> (w436:dbl)
                n281 = Not Equal?(x=w434, y=w436) -> (x != y?=w435:bool)
                n282 = case shown="True" w435 {
                  tunnel: w434 -> [_ w437]
                  frame False {
                  }
                  frame True {
                    n283 = property on="Wavelength" class="DigNum (strict)"("Val(Sgnl)"=w437) -> ()  [unwired: 2 in, 2 out]
                  }
                }
              }
            }
            n284 = local read "State next step"() -> (w300:string)
            "queue #" <- w299
          }
          frame "Walker" {
            w444 = dbl[] [680.0, 730.0, 780.0, 830.0, 880.0, 930.0, 980.0, 1030.0, 980.0, 930.0, 880.0, 830.0, 780.0, 730.0, 680.0, 800.0] ("Array")
            n285 = Wait (ms)(milliseconds to wait=2000) -> ()  [unwired: 1 out]
            n286 = local read "Step"() -> (w446:dbl)
            n287 = Index Array(array=w444, index=w446) -> (element=w440:dbl)
            n288 = Array Size(array=w444) -> (size(s)=w443:i32)
            n289 = Increment(x=w446) -> (x+1=w442:dbl)
            n290 = property on="Wavelength" class="DigNum (strict)"("Val(Sgnl)"=w440) -> ()  [unwired: 2 in, 2 out]
            n291 = Equal?(x=w442, y=w443) -> (x = y?=w441:bool)
            n292 = case shown="True" w441 {
              tunnel: w442 -> [w449 _]
              tunnel: [TRUE FALSE ("Walking")] -> w439
              frame False {
                n293 = local write "Step"(w449) -> ()
              }
              frame True {
                n294 = local write "WV Walk"(FALSE) -> ()
                n295 = local write "State next step"("Writer") -> ()
              }
            }
            "Walking" <- w439
          }
          frame "Backuper" {
            n296 = local read "Backuper state"() -> (w454:string)
            n297 = case shown="\"BackupFinal\"" w454 {
              tunnel: w456 -> [_ w479]
              frame "BackupInit", Default {
                n298 = flat-sequence {
                  frame #0 {
                    n299 = Wait (ms)(milliseconds to wait=u32 30000) -> ()  [unwired: 1 out]
                    n300 = local write "Backuper state"("BackupFinal") -> ()
                  }
                  frame #1 {
                    n301 = local write "Refresh"(TRUE ("Refresh")) -> ()
                  }
                }
              }
              frame "BackupFinal" {
                n302 = local write "Backup"(FALSE ("Backup")) -> ()
                n303 = local write "State next step"("Writer") -> ()
                n304 = local write "Backuper state"("BackupInit") -> ()
                n305 = local read "SavePath"() -> (w460:path)
                n306 = String To IP() -> (0:w473:u32)  [unwired: 1 in]
                n307 = IP To String(2:w473) -> (0:w461:string)  [unwired: 1 in]
                n308 = call "create unique folder.vi"("string"=w461, "path 2"=w460) -> ("path"=w466:path)  [unwired: 9 in]
                n309 = Get Date/Time In Seconds() -> (seconds since 1Jan1904=w475:timestamp)
                n310 = Format Date/Time String(time format string (%c)="%Y-%m-%d-%H-%M-%S", seconds (now)=w475) -> (date/time string=w470:string)  [unwired: 1 in]
                n311 = Path To String(path=w466) -> (string=w472:string)
                n312 = Concatenate Strings(w472, "\\" ("string"), w470, ".csv" ("string")) -> (w469:string)
                n313 = String To Path(string=w469) -> (path=w468:path)
                n314 = call-poly <vilib>:"Write To Spreadsheet File.vi"("delimiter (\\t)"="," ("delimiter (\\t)"), "format (%s)"="%.6f" ("format (%.3f)"), "append to file? (new file:F)"=FALSE, "2D data"=w479, "file path (dialog if empty)"=w468) -> ()  [unwired: 2 in, 2 out]
                "Backing up" <- FALSE ("Backing up ...")
              }
            }
          }
          frame "Quiter" {
            n315 = Equal To 0?(x=w484) -> (x = 0?=w483:bool)
            n316 = case shown="True" w483 {
              tunnel: ["Quiter" "Writer"] -> w482
              tunnel: [FALSE w488] -> w481
              frame False {
              }
              frame True {
                n317 = local read "Sleep"() -> (w487:bool)
                n318 = case shown="True" w487 {
                  tunnel: [w491 _] -> w488
                  frame False {
                    n319 = local read "QUIT"() -> (w490:bool)
                    n320 = case shown="True" w490 {
                      tunnel: [_ w492] -> w491
                      frame False {
                      }
                      frame True {
                        w492 = TRUE
                        n321 = local write "QUIT"(FALSE) -> ()
                        n322 = local write "stop"(w492) -> ()
                      }
                    }
                  }
                  frame True {
                    w494 = FALSE ("Sleep")
                    n323 = property on="Laser Control" class="Bool (strict)"("Val(Sgnl)"=w494) -> ()  [unwired: 2 in, 2 out]
                    n324 = local write "Sleeping"(w494) -> ()
                    n325 = local write "Sleep"(w494) -> ()
                    n326 = local write "State next step"("Writer" ("State next step")) -> ()
                  }
                }
              }
            }
          }
        }
      }
      n327 = VISA Close(VISA resource name=w58, error in (no error)=w57) -> (error out=w63:errorcluster)
      n328 = call <vilib>:"Simple Error Handler.vi"("error in (no error)"=w63) -> ()  [unwired: 1 in, 8 out]
    }
  }
